vi "Open Shutter.vi"(8 "error in (no error)":errorcluster, 10 "Open Shutter":bool, 11 "Topas in":refnum<class "Topas.lvclass">) -> (0 "error out":errorcluster, 3 "Topas out":refnum<class "Topas.lvclass">)   [LabVIEW 2019, in "Topas.lvclass"]
uses:
  Topas.lvclass
  Topas.lvclass/Topas.ctl
  Topas-LabVIEW-Driver/TopasDriver.lvlib
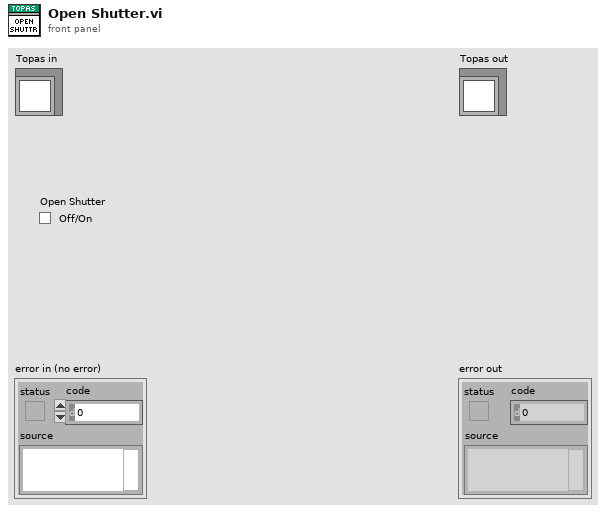
[diagram p1: front panel]
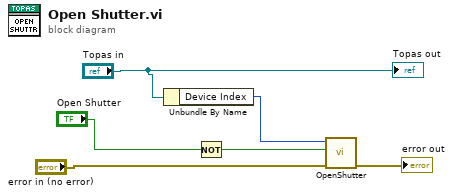
[diagram p0: block diagram]
diagram:
  n1 = Unbundle By Name("Topas in") -> ("Device Index"=w1:u8)
  n2 = Not(x="Open Shutter") -> (.not. x?=w3:bool)
  n3 = call "OpenShutter.vi"("error in (no error)"="error in (no error)", "Open Shutter"=w3, "Device Index"=w1) -> ("error out"=→"error out":errorcluster)  [unwired: 7 in, 1 out]
  "Topas out" <- "Topas in"
